vi "arduino1ledonoff.vi"() -> ()   [LabVIEW 2015]
uses:
  <vilib>/LabVIEW Interface for Arduino/Type Defs/Pin Mode.ctl
  <vilib>/LabVIEW Interface for Arduino/LabVIEW Interface for Arduino.lvlib
panel:
  in  "stop":bool
  in  "Boolean":bool
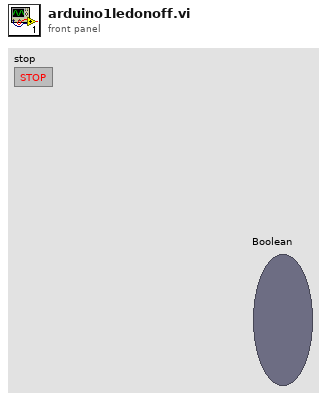
[diagram p1: front panel]
types:
  T1 = typedef "LabVIEW Interface for Arduino.lvlib/Pin Mode.ctl" = enum8{"Input", "Output"}
  T2 = typedef "LabVIEW Interface for Arduino.lvlib/Arduino Resource.ctl" = cluster{"VISA resource":refnum<visa-resource-name>, "Board Type":T3, "Connection Type":enum8{"USB / Serial"}, "Bytes Per Packet (15)":u8}
  T3 = typedef "LabVIEW Interface for Arduino.lvlib/Board Type.ctl" = enum16{"Uno", "Dimuelanove w/Atmega 328", "Mega 2560"}
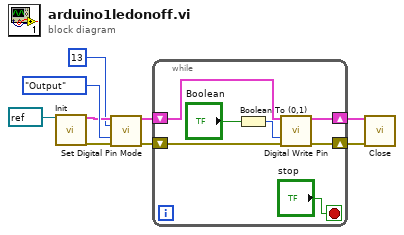
[diagram p0: block diagram]
diagram:
  n1 = call <vilib>:"Init.vi"("VISA resource"=refnum<visa-resource-name> refnum) -> ("Arduino Resource"=w6:T2, "error out"=w3:errorcluster)  [unwired: 17 in]
  n2 = call <vilib>:"Set Digital Pin Mode.vi"("Arduino Resource"=w6, "Digital I/O Pin"=u8 13, "Pin Mode (Input)"=Pin_Mode."Output", "error in"=w3) -> ("Arduino Resource"=w5:T2, "error out"=w4:errorcluster)  [unwired: 10 in]
  n3 = while {
    shift-right: [w16] -> w8
    shift-left: w5 -> [w15]
    shift-right: [w14] -> w9
    shift-left: w4 -> [w10]
    stop <- "stop" stop-if-true
    n4 = Boolean To (0,1)(Boolean="Boolean") -> (0, 1=w12:i16)
    n5 = call <vilib>:"Digital Write Pin.vi"("Arduino Resource"=w15, "Value (0)"=w12, "error in"=w10) -> ("Arduino Resource"=w16:T2, "error out"=w14:errorcluster)  [unwired: 11 in]
  }
  n6 = call <vilib>:"Close.vi"("Arduino Resource"=w8, "error in"=w9) -> ()  [unwired: 13 in, 1 out]
